vi "RFmx MP Apply DPD.vi"(0 "Instrument Handle In":refnum<k21>, 1 "Selector String":string, 5 "RFSG handle":refnum<k15>, 7 "RFmx DPD Common Configuration":T4={"DPD Measurement Interval (s)"=0.0001, "Sample Rate Mode"=1, "Sample Rate (S/s)"=120000000.0, "Signal Type"=0, "Pre DPD CFR Enabled"=0, "Apply DPD CFR Enabled"=0, "DUT Average Input Power (dBm)"=-15.0} {"DUT Average Input Power (dBm)" format="%.2f"; "Apply DPD CFR Enabled" items=["False", "True"]; "Pre DPD CFR Enabled" items=["False", "True"]; "Signal Type" items=["Modulated", "Tones"]; "Sample Rate (S/s)" format="%.2p"; "Sample Rate Mode" items=["User", "Reference Waveform"]; "DPD Measurement Interval (s)" format="%#.2p"}, 9 "Waveform":T1={"Waveform Name"="Wfm", "Waveform"={"x0"=0.0, "dx"=0.0, "y"=[]}, "Signal Bandwidth (Hz)"=0.0, "PAPR (dB)"=0.0, "Burst Length (s)"=0.0, "Sample Rate"=0.0, "Burst Start Locations"=[], "Burst Stop Locations"=[], "Idle Duration Present?"=FALSE, "Runtime Scaling"=0.0} {"Runtime Scaling" format="%#_6p"; "Sample Rate" format="%#_6p"; "Burst Length (s)" format="%#_6p"; "PAPR (dB)" format="%.2f"; "Signal Bandwidth (Hz)" format="%#_6p"; "Waveform"."y" format="%.2f"; "Waveform"."dx" format="%^.2e"; "Waveform"."x0" format="%^.2e"}, 11 "error in (no error)":errorcluster) -> (4 "Instrument Handle Out":refnum<k21>, 6 "RFSG instrument handle out":refnum<k15>, 8 "RFmx MP Results":T2={"Waveform Out"={"x0"=0.0, "dx"=0.0, "y"=[]}, "Post DPD PAPR (dB)"=-1.0, "Power Offset (dB)"=-1.0, "DPD Polynomial"=[]} {"DPD Polynomial" format="%.2f"; "Power Offset (dB)" format="%.2f"; "Post DPD PAPR (dB)" format="%.2f"; "Waveform Out"."y" format="%.2f"; "Waveform Out"."dx" format="%^.2e"; "Waveform Out"."x0" format="%^.2e"}, 15 "error out":errorcluster)   [LabVIEW 2018, in "DPD.lvlib"]
uses:
  DPD.lvlib
  Typedefs/RFmx DPD Common Configuration.ctl
  Typedefs/Rfmx MP Configuration.ctl
  Typedefs/RFmx MP Results.ctl
  SG/Typedefs/Waveform.ctl
  <vilib>/RFmx/SpecAn/mx/RFmxSpecAn.llb/RFmxSpecAn DPD Fetch DPD Polynomial.vi
  SG/SG.lvlib
panel:
  in  "RFmx MP Configuration":T3={"Mem Models Correction Type"=0, " Iterative DPD Enabled"=0, "Number of Iterations"=3, "Polynomial  Order"=3, "Memory Depth"=2, "Maximum Lag"=2, "Maximum Lead"=2, "Lag Order"=2, "Lead Order"=2, "Lag Memory Depth"=2, "Lead Memory Depth"=2} {"Number of Iterations" min=1; "Iterative DPD Enabled" items=["False", "True"]; "Mem Models Correction Type" items=["Magnitude and Phase", "Magnitude Only", "Phase Only"]}
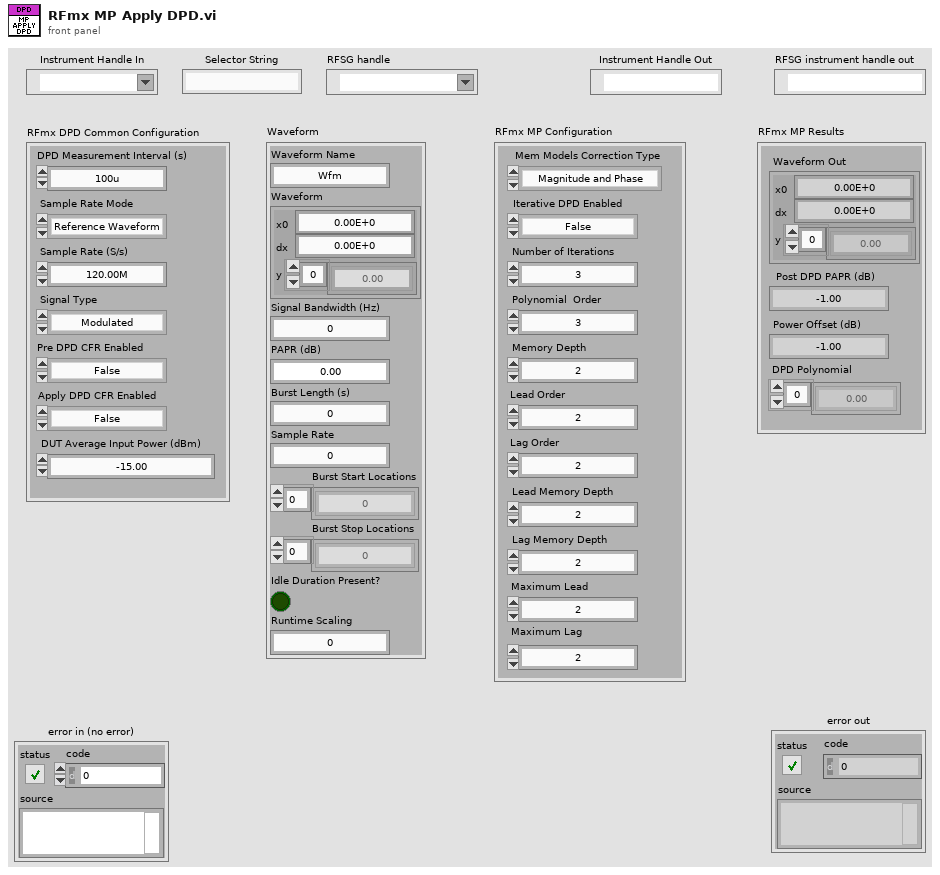
[diagram p1: front panel]
types:
  T1 = typedef "SG.lvlib/Waveform.ctl" = cluster{"Waveform Name":string, "Waveform":cluster{"x0":dbl, "dx":dbl, "y":csg[]}, "Signal Bandwidth (Hz)":dbl, "PAPR (dB)":dbl, "Burst Length (s)":dbl, "Sample Rate":dbl, "Burst Start Locations":i32[], "Burst Stop Locations":i32[], "Idle Duration Present?":bool, "Runtime Scaling":dbl}
  T2 = typedef "DPD.lvlib/RFmx MP Results.ctl" = cluster{"Waveform Out":cluster{"x0":dbl, "dx":dbl, "y":csg[]}, "Post DPD PAPR (dB)":dbl, "Power Offset (dB)":dbl, "DPD Polynomial":csg[]}
  T3 = typedef "DPD.lvlib/Rfmx MP Configuration.ctl" = cluster{"Mem Models Correction Type":i32, " Iterative DPD Enabled":i32, "Number of Iterations":i32, "Polynomial  Order":i32, "Memory Depth":i32, "Maximum Lag":i32, "Maximum Lead":i32, "Lag Order":i32, "Lead Order":i32, "Lag Memory Depth":i32, "Lead Memory Depth":i32}
  T4 = typedef "DPD.lvlib/RFmx DPD Common Configuration.ctl" = cluster{"DPD Measurement Interval (s)":dbl, "Sample Rate Mode":i32, "Sample Rate (S/s)":dbl, "Signal Type":i32, "Pre DPD CFR Enabled":i32, "Apply DPD CFR Enabled":i32, "DUT Average Input Power (dBm)":dbl}
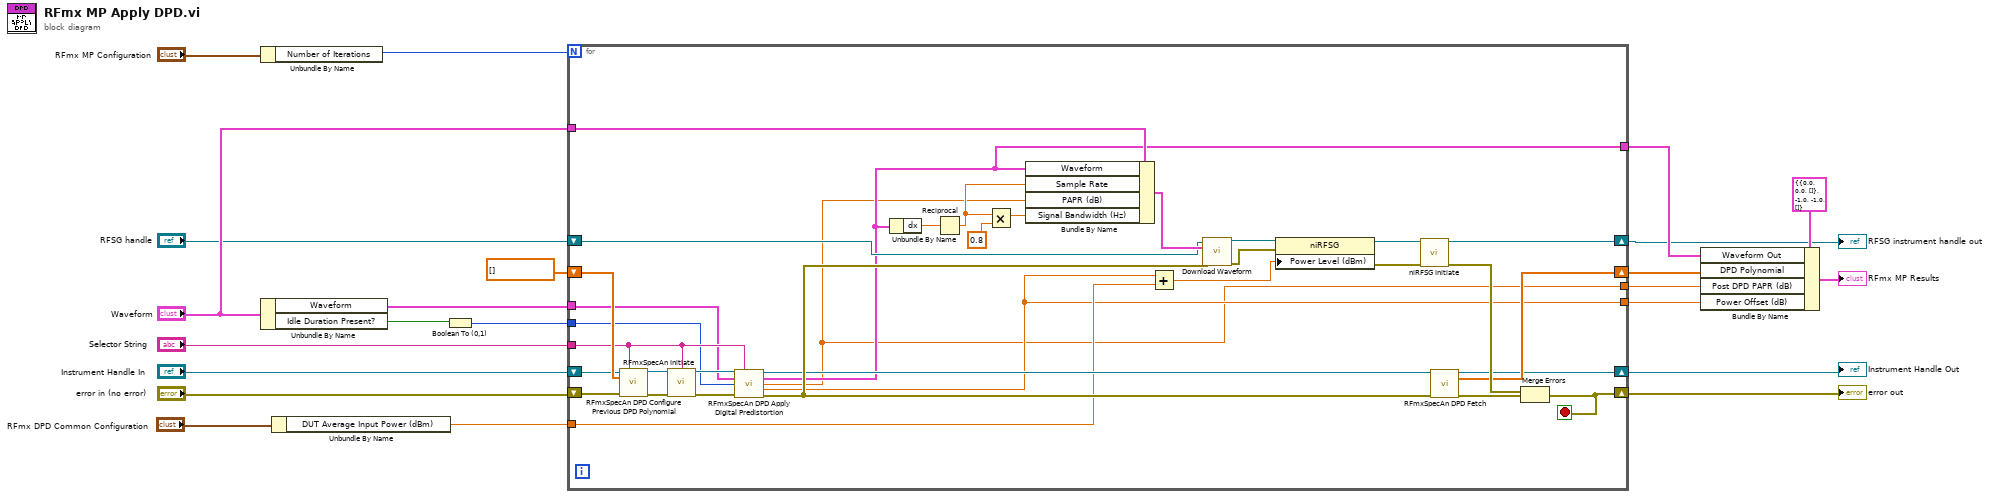
[diagram p0: block diagram]
diagram:
  n1 = Unbundle By Name("RFmx MP Configuration") -> ("Number of Iterations"=w10:i32)
  n2 = Unbundle By Name("Waveform") -> ("Waveform"=w16:cluster{"x0":dbl, "dx":dbl, "y":csg[]}, "Idle Duration Present?"=w18:bool)
  n3 = Unbundle By Name("RFmx DPD Common Configuration") -> ("DUT Average Input Power (dBm)"=w14:dbl)
  n4 = Boolean To (0,1)(Boolean=w18) -> (0, 1=w17:i16)
  n5 = for {
    N: w10 -> [_]
    shift-right: [w23] -> w2
    shift-left: "Instrument Handle In" -> [w39]
    shift-right: [w56] -> w7
    shift-left: "error in (no error)" -> [w38]
    shift-right: [w27] -> w9
    shift-left: csg[] [] ("DPD Polynomial") -> [w54]
    tunnel: "Selector String" -> [w37]
    tunnel: w17 -> [w36]
    tunnel: w16 -> [w35]
    tunnel: w14 -> [w32]
    tunnel: "Waveform" -> [w31]
    shift-right: [w28] -> w1
    shift-left: "RFSG handle" -> [w29]
    tunnel: [w26] -> w8
    tunnel: [w25] -> w4
    tunnel: [w24] -> w3
    stop <- w56 stop-if-true
    n6 = call <vilib>:"RFmxSpecAn DPD Configure Previous DPD Polynomial.vi"("Instrument Handle In"=w39, "Selector String"=w37, "Previous DPD Polynomial"=w54, "error in (no error)"=w38) -> ("Instrument Handle Out"=w52:refnum<k21>, "error out"=w53:errorcluster)  [unwired: 10 in]
    n7 = call <vilib>:"RFmxSpecAn Initiate.vi"("Instrument Handle In"=w52, "Result Name"=w37, "error in (no error)"=w53) -> ("Instrument Handle Out"=w43:refnum<k21>, "error out"=w42:errorcluster)  [unwired: 10 in, 1 out]
    n8 = call <vilib>:"RFmxSpecAn DPD Apply Digital Predistortion.vi"("Instrument Handle In"=w43, "Selector String"=w37, "Waveform In"=w35, "Idle Duration Present"=w36, "error in (no error)"=w42) -> ("Instrument Handle Out"=w34:refnum<k21>, "Waveform Out"=w26:cluster{"x0":dbl, "dx":dbl, "y":csg[]}, "PAPR (dB)"=w24:dbl, "Power Offset (dB)"=w25:dbl, "error out"=w41:errorcluster)  [unwired: 6 in]
    n9 = Unbundle By Name(w26) -> ("dx"=w44:dbl)
    n10 = Reciprocal(x=w44) -> (1/x=w45:dbl)
    n11 = Multiply(x=w45, y=0.8) -> (x*y=w46:dbl)
    n12 = Bundle By Name(cluster=w31, "Waveform"=w26, "Sample Rate"=w45, "PAPR (dB)"=w24, "Signal Bandwidth (Hz)"=w46) -> (w30:T1)
    n13 = Add(x=w25, y=w32) -> (x+y=w49:dbl)
    n14 = call "Download Waveform.vi"("RFSG handle"=w29, "Waveform In"=w30, "error in (no error)"=w41) -> ("RFSG handle out"=w47:refnum<k15>, "error out"=w48:errorcluster)  [unwired: 11 in]
    n15 = property class="niRFSG"(reference=w47, error in=w48, "Power Level (dBm)"=w49) -> (reference out=w50:refnum<k15>, error out=w51:errorcluster)
    n16 = call <instrlib>:"niRFSG Initiate.vi"("instrument handle"=w50, "error in"=w51) -> ("instrument handle out"=w28:refnum<k15>, "error out"=w40:errorcluster)  [unwired: 12 in]
    n17 = call-poly <vilib>:"RFmxSpecAn DPD Fetch.vi"("Instrument Handle In"=w34, "error in (no error)"=w41) -> ("Instrument Handle Out"=w23:refnum<k21>, "DPD Polynomial"=w27:csg[], "error out"=w55:errorcluster)  [unwired: 11 in]
    n18 = Merge Errors(w40, w55) -> (w56:errorcluster)
  }
  "error out" <- w7
  "Instrument Handle Out" <- w2
  "RFSG instrument handle out" <- w1
  n19 = Bundle By Name(cluster=T2 {"Waveform Out"={"x0"=0.0, "dx"=0.0, "y"=[]}, "Post DPD PAPR (dB)"=-1.0, "Power Offset (dB)"=-1.0, "DPD Polynomial"=[]} ("RFmxMP Results"), "Waveform Out"=w8, "DPD Polynomial"=w9, "Post DPD PAPR (dB)"=w3, "Power Offset (dB)"=w4) -> (→"RFmx MP Results":T2)
